vi "Read File of SubFolders_ElemByElem.vi"(8 "error in (no error)":errorcluster, 10 "indices":i32[](array[numeric]), 11 "Folder_Mgmt in":refnum<class "Folder_Mgmt.lvclass">) -> (0 "error out":errorcluster, 2 "?":string, 3 "Folder_Mgmt out":refnum<class "Folder_Mgmt.lvclass">)   [LabVIEW 2016, in "Folder_Mgmt.lvclass"]
uses:
  Folder_Mgmt.lvclass
  Folder_Mgmt.lvclass/Folder_Mgmt.ctl
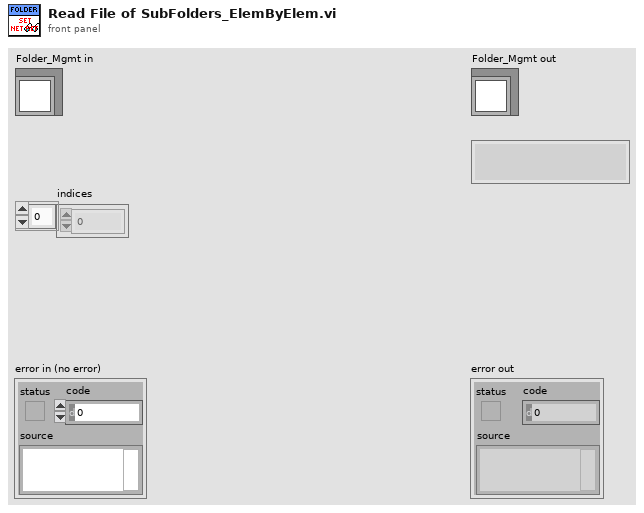
[diagram p1: front panel]
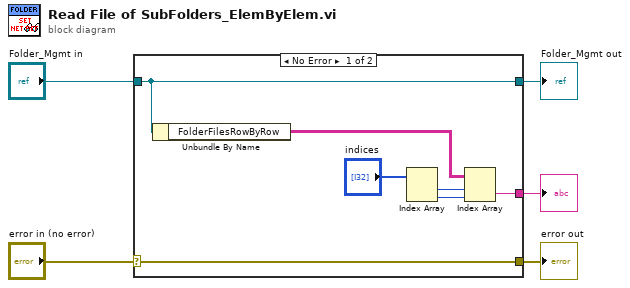
[diagram p0: block diagram]
diagram:
  n1 = case shown="No Error" "error in (no error)" {
    selector: "error in (no error)" -> [w12 w13]
    tunnel: [w12 w13] -> w4
    tunnel: [w11 w14] -> w2
    tunnel: "Folder_Mgmt in" -> [w11 w14]
    tunnel: [w10 _] -> w1
    frame No Error {
      n2 = Unbundle By Name(w11) -> ("FolderFilesRowByRow"=w6:string[][])
      n3 = Index Array(array="indices") -> (element #1=w8:i32, element #2=w7:i32)  [unwired: 2 in]
      n4 = Index Array(array=w6, index (row)=w8, index (col)=w7) -> (element=w10:string)
    }
    frame Error {
    }
  }
  "error out" <- w4
  "Folder_Mgmt out" <- w2
  "?" <- w1
